vi "Close Module.vi"(8 "error in (no error)":errorcluster, 9 "Wait for stop?":bool, 11 "Module Admin in":refnum<class "Delacor_lib_QMH_Cloneable Module Admin.lvclass">) -> (0 "error out":errorcluster, 1 "External Launch":bool, 3 "Module Admin out":refnum<class "Delacor_lib_QMH_Cloneable Module Admin.lvclass">)   [LabVIEW 2020, in "GenNet-Server.lvlib"]
doc: "Destroy the Broadcast Events and Request Events (if this was the first instance). Reset flags stored in Module Admin class.\n____\nHAMPEL SOFTWARE ENGINEERING v3.8.0 (2023-12-18 14:41)"
uses:
  GenNet-Server.lvlib
  <vilib>/Delacor/Delacor QMH/Libraries/Cloneable Module Admin_class/Delacor_lib_QMH_Cloneable Module Admin.lvclass
  C:/Program Files (x86)/National Instruments/LabVIEW 2020/vi.lib/Delacor/Delacor QMH/Libraries/Module Admin_class/Delacor_lib_QMH_Module Admin.lvclass
  Stop Argument--cluster.ctl
  <vilib>/Delacor/Delacor QMH/Libraries/Cloneable Module Admin_class/Delacor_lib_QMH_Cloneable Module Admin.lvclass/Delacor_lib_QMH_Cloneable Module Admin.ctl
  <vilib>/Delacor/Delacor QMH/Libraries/Module Admin_class/Delacor_lib_QMH_Module Admin.lvclass/Delacor_lib_QMH_Module Admin.ctl
  <vilib>/Delacor/Delacor QMH/Libraries/Cloneable Module Admin_class/Delacor_lib_QMH_Get First.vi
  <vilib>/Delacor/Delacor QMH/Libraries/Cloneable Module Admin_class/Delacor_lib_QMH_Get Module ID.vi
  <vilib>/Delacor/Delacor QMH/Libraries/Module Admin_class/Delacor_lib_QMH_Get External Launch.vi
  <vilib>/Delacor/Delacor QMH/Libraries/Cloneable Module Admin_class/Delacor_lib_QMH_Get Close Master Reference.vi
  Clone Registration/Clone Registration.lvlib
  VI Reference Management/VI Reference Management.lvlib
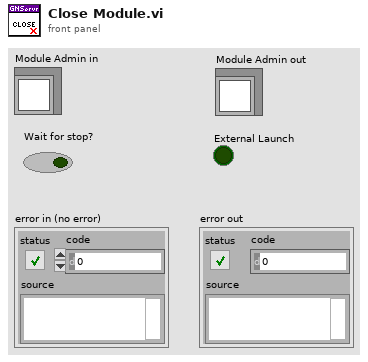
[diagram p1: front panel]
types:
  T1 = typedef "GenNet-Server.lvlib/Stop Argument--cluster.ctl" = cluster{"Origin":string, "Module ID":i32, "Exit via Stop Module Req?":bool, "Wait for Module to stop?":bool}
  T2 = typedef "Semaphore RefNum" = refnum<k1>
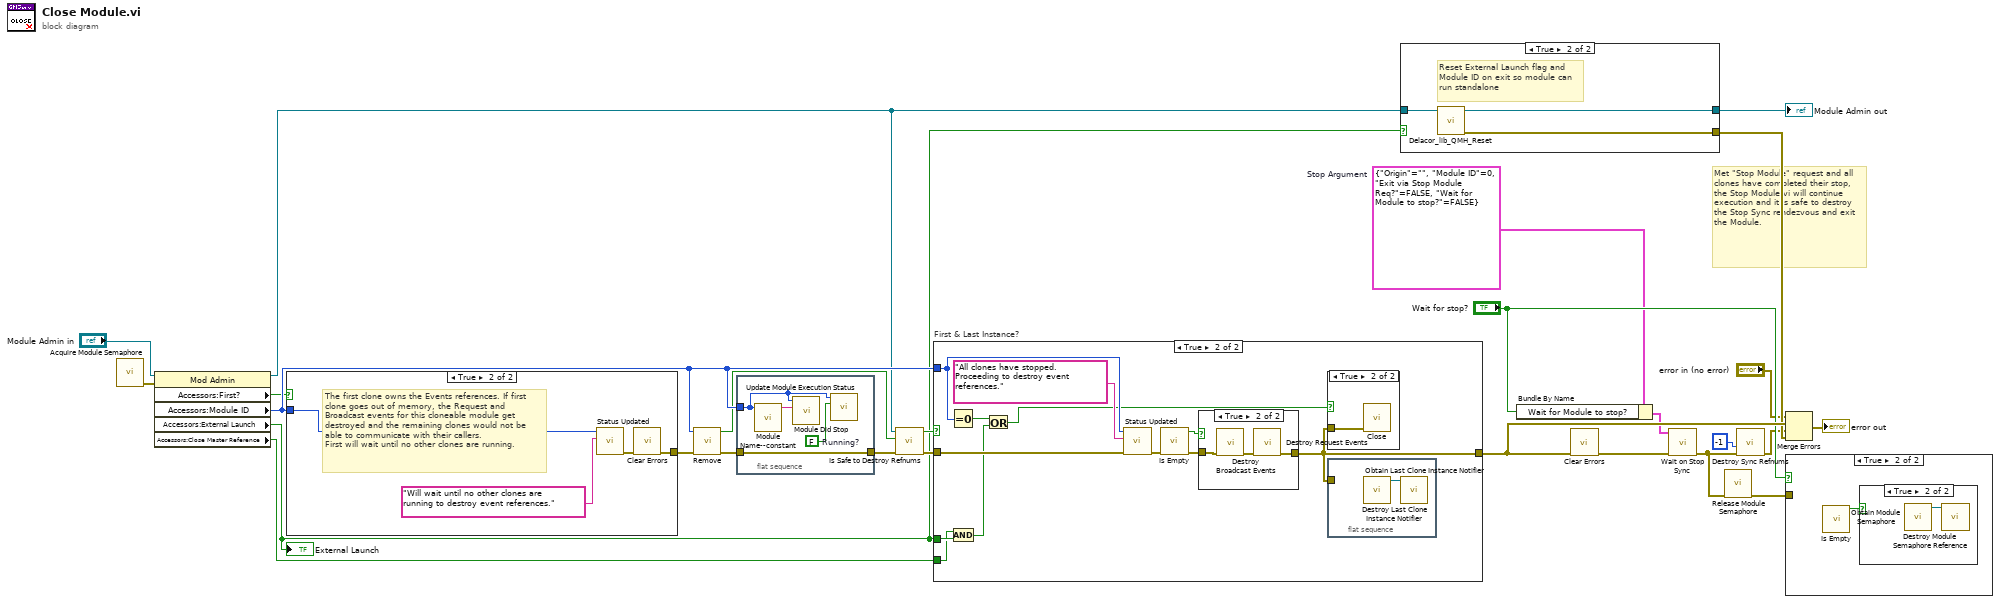
[diagram p0: block diagram]
diagram:
  w2 = T1 {"Origin"="", "Module ID"=0, "Exit via Stop Module Req?"=FALSE, "Wait for Module to stop?"=FALSE}  # Stop Argument
  # "Met \"Stop Module\" request and all clones have completed their stop, the Stop Module.vi will continue execution and it is safe to destroy the Stop Sync rendezvous and exit the Module."
  n1 = call "Acquire Module Semaphore.vi"() -> ("error out"=w5:errorcluster)  [unwired: 11 in]
  n2 = property on="Property Node" class="Mod Admin"(reference="Module Admin in", error in=w5) -> (reference out=w21:refnum<class "Delacor_lib_QMH_Cloneable Module Admin.lvclass">, "Accessors:First?"=w11:bool, "Accessors:Module ID"=w25:i32, "Accessors:External Launch"=w7:bool, "Accessors:Close Master Reference"=w6:bool)  [unwired: 1 out]
  "External Launch" <- w7
  n3 = case shown="True" w11 {
    tunnel: w25 -> [_ w29]
    tunnel: [_ w27] -> w26
    frame False {
    }
    frame True {
      # "The first clone owns the Events references. If first clone goes out of memory, the Request and Broadcast events for this cloneable module get destroyed and the remaining clones would not be able to communicate with their callers.\nFirst will wait until no other clones are running."
      n4 = call "Status Updated.vi"("Status"="Will wait until no other clones are running to destroy event references." ("format string"), "Module ID"=w29) -> ("error out"=w28:errorcluster)  [unwired: 9 in]
      n5 = call <vilib>:"Clear Errors.vi"("error in (no error)"=w28) -> ("error out"=w27:errorcluster)  [unwired: 5 in, 1 out]
    }
  }
  n6 = call "Remove.vi"("error in (no error)"=w26, "Module ID"=w25) -> ("error out"=w22:errorcluster, "empty"=w9:bool)  [unwired: 7 in, 1 out]
  n7 = flat-sequence {
    tunnel: w22 -> [w34]
    tunnel: [w34] -> w8
    tunnel: w25 -> [w32]
    frame #0 {
      w31 = FALSE  # Running?
      n8 = call "Module Name--constant.vi"("Module ID"=w32) -> ("Module Name"=w33:string)  [unwired: 10 in]
      n9 = call "Module Did Stop.vi"("Origin"=w33, "Module ID"=w32) -> ()  [unwired: 9 in, 1 out]
      n10 = call "Update Module Execution Status.vi"("Running?"=w31, "Module ID"=w32) -> ()  [unwired: 9 in, 1 out]
    }
  }
  n11 = call "Is Safe to Destroy Refnums.vi"("error in (no error)"=w8, "empty"=w9, "Module Admin"=w21) -> ("error out"=w18:errorcluster, "Destroy Broadcast & Request Event Refs?"=w19:bool)  [unwired: 7 in]
  n12 = case "First & Last Instance?" shown="True" w19 {
    tunnel: w18 -> [w35 w47]
    tunnel: [w35 w43] -> w24
    tunnel: w25 -> [_ w46]
    tunnel: w7 -> [_ w40]
    tunnel: w6 -> [_ w39]
    frame False {
    }
    frame True {
      n13 = Equal To 0?(x=w46) -> (x = 0?=w38:bool)
      n14 = And(x=w39, y=w40) -> (x .and. y?=w36:bool)
      n15 = Or(x=w38, y=w36) -> (x .or. y?=w37:bool)
      n16 = call "Status Updated.vi"("error in (no error)"=w47, "Status"="All clones have stopped. Proceeding to destroy event references.", "Module ID"=w46) -> ("error out"=w44:errorcluster)  [unwired: 8 in]
      n17 = call "Is Empty.vi"("error in (no error)"=w44) -> ("error out"=w41:errorcluster, "Empty?"=w42:bool)  [unwired: 9 in]
      n18 = case shown="True" w42 {
        tunnel: w41 -> [w49 w52]
        tunnel: [w49 w50] -> w43
        frame False {
        }
        frame True {
          n19 = call "Destroy Broadcast Events.vi"("error in (no error)"=w52) -> ("error out"=w51:errorcluster)  [unwired: 10 in]
          n20 = call "Destroy Request Events.vi"("error in (no error)"=w51) -> ("error out"=w50:errorcluster)  [unwired: 10 in]
        }
      }
      n21 = case shown="True" w37 {
        tunnel: w43 -> [_ w48]
        frame False {
        }
        frame True {
          n22 = call "Close.vi"("error in (no error)"=w48) -> ()  [unwired: 10 in, 1 out]
        }
      }
      n23 = flat-sequence {
        tunnel: w43 -> [_]
        frame #0 {
          n24 = call "Obtain Last Clone Instance Notifier.vi"() -> ("Last Instance Notifier"=w53:refnum<notifier>)  [unwired: 10 in, 1 out]
          n25 = call "Destroy Last Clone Instance Notifier.vi"("Last Instance Notifier"=w53) -> ()  [unwired: 11 in]
        }
      }
    }
  }
  n26 = case shown="True" w7 {
    tunnel: w21 -> [w54 w57]
    tunnel: [w54 w56] -> w17
    tunnel: [_ w55] -> w23
    frame False {
    }
    frame True {
      # "Reset External Launch flag and Module ID on exit so module can run standalone"
      n27 = call-dynamic "Delacor_lib_QMH_Reset.vi"("Mod Admin in"=w57) -> ("error out"=w55:errorcluster, "Mod Admin out"=w56:refnum<class "Delacor_lib_QMH_Cloneable Module Admin.lvclass">)  [unwired: 9 in]
    }
  }
  "Module Admin out" <- w17
  n28 = Bundle By Name(cluster=w2, "Wait for Module to stop?"="Wait for stop?") -> (w1:T1)
  n29 = call <vilib>:"Clear Errors.vi"("error in (no error)"=w24) -> ("error out"=w13:errorcluster)  [unwired: 5 in, 1 out]
  n30 = call "Wait on Stop Sync.vi"("error in"=w13, "Stop Argument"=w1) -> ("error out"=w3:errorcluster)  [unwired: 9 in]
  n31 = call "Release Module Semaphore.vi"("error in (no error)"=w3) -> ("error out"=w4:errorcluster)  [unwired: 10 in]
  n32 = call "Destroy Sync Refnums.vi"("error in (no error)"=w3, "Module ID"=-1) -> ("error out"=w15:errorcluster)  [unwired: 9 in]
  n33 = Merge Errors("error in (no error)", w24, w15, w23) -> (→"error out":errorcluster)
  n34 = case shown="True" "Wait for stop?" {
    tunnel: w4 -> [_ _]
    frame False {
    }
    frame True {
      n35 = call "Is Empty.vi"() -> ("Empty?"=w58:bool)  [unwired: 10 in, 1 out]
      n36 = case shown="True" w58 {
        frame False {
        }
        frame True {
          n37 = call "Obtain Module Semaphore.vi"() -> ("semaphore"=w59:T2)  [unwired: 9 in, 2 out]
          n38 = call "Destroy Module Semaphore Reference.vi"("semaphore"=w59) -> ()  [unwired: 10 in, 1 out]
        }
      }
    }
  }
